vi "ConfigArbWfrm.vi"(8 "error in (no error)":errorcluster, 11 "ClassIn":refnum<class "NiPxi6733.lvclass">) -> (0 "error out":errorcluster, 3 "ClassOut":refnum<class "NiPxi6733.lvclass">)   [LabVIEW 2014, in "FGenPlugins.lvlib" / "NiPxi6733.lvclass"]
uses:
  NiPxi6733.lvclass
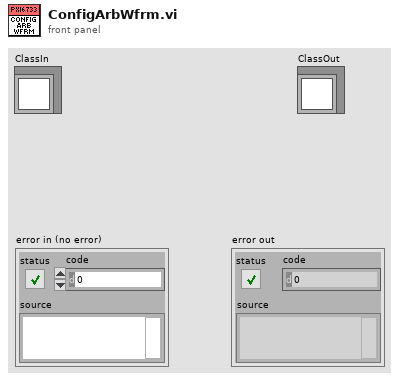
[diagram p1: front panel]
types:
  T1 = typedef "NISTFGenPlugins.lvlib/NISTFGenPluginsBase.lvclass/ArbWfrmParams.ctl" = cluster{"sWfrmHandle":string, "iSize":i32, "dData":dbl[], "dGain":dbl, "dOffset":dbl, "dSampleRate":dbl}
  T2 = typedef "FGenPlugins.lvlib/NISTFGenPluginsBase.lvclass/ChannelParamElement.ctl" = cluster{"sName":string, "eOperateMode":u16, "bEnabled":bool, "eOutputMode":u16, "iIndex":i32, "iNameBufferSize":i32, "fGain":dbl}
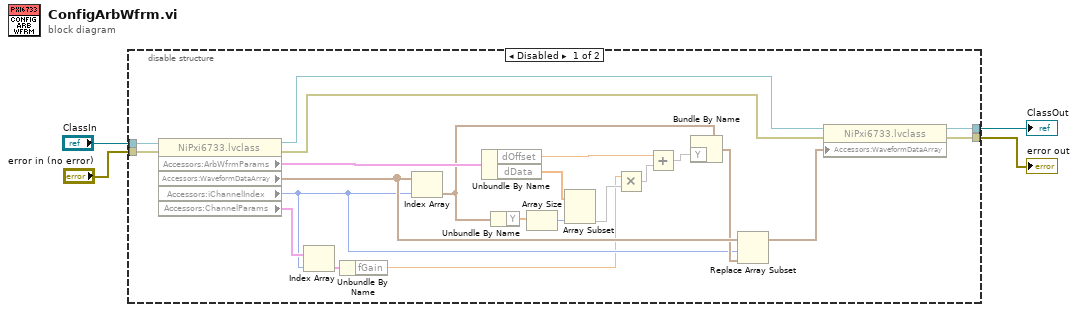
[diagram p0: block diagram]
diagram:
  n1 = disable-structure shown="Disabled" {
    disable-tunnel: "ClassIn" -> [w26 w28]
    disable-tunnel: "error in (no error)" -> [w25 w27]
    disable-tunnel: [w24 w28] -> w2
    disable-tunnel: [w23 w27] -> w1
    frame Disabled {
      n2 = property class="NiPxi6733.lvclass"(reference=w26, error in=w25) -> (reference out=w17:refnum<class "NiPxi6733.lvclass">, error out=w9:errorcluster, "Accessors:ArbWfrmParams"=w19:T1, "Accessors:WaveformDataArray"=w16:waveform(dbl)[], "Accessors:iChannelIndex"=w7:i32, "Accessors:ChannelParams"=w8:T2[])
      n3 = Index Array(array=w8, index=w7) -> (element=w6:T2)
      n4 = Unbundle By Name(w6) -> ("fGain"=w5:dbl)
      n5 = Index Array(array=w16, index=w7) -> (element=w18:waveform(dbl))
      n6 = Unbundle By Name(w19) -> ("dOffset"=w22:dbl, "dData"=w12:dbl[])
      n7 = Unbundle By Name(w18) -> ("Y"=w13:dbl[])
      n8 = Array Size(array=w13) -> (size(s)=w11:i32)
      n9 = Array Subset(array=w12, length=w11) -> (w10:dbl[])  [unwired: 1 in]
      n10 = Multiply(x=w5, y=w10) -> (x*y=w21:dbl[])
      n11 = Add(x=w22, y=w21) -> (x+y=w20:dbl[])
      n12 = Bundle By Name(cluster=w18, "Y"=w20) -> (w15:waveform(dbl))
      n13 = Replace Array Subset(array=w16, new element=w15, index=w7) -> (w14:waveform(dbl)[])
      n14 = property class="NiPxi6733.lvclass"(reference=w17, error in=w9, "Accessors:WaveformDataArray"=w14) -> (reference out=w24:refnum<class "NiPxi6733.lvclass">, error out=w23:errorcluster)
    }
    frame Enabled {
    }
  }
  "error out" <- w1
  "ClassOut" <- w2
